vi "Get Angler Position Arrays.vi"(11 "Position Array":T1[](array[typedef])=[{"Angle"=1.0, "Count"=47}, {"Angle"=6.0, "Count"=213}, {"Angle"=5.0, "Count"=383}, {"Angle"=4.0, "Count"=557}, {"Angle"=3.0, "Count"=724}, {"Angle"=2.0, "Count"=898}]) -> (2 "Position Array":i32[](array[numeric]), 3 "Angle Array":dbl[](array[numeric]))   [LabVIEW 2023, in "Angler_ACT.lvlib"]
uses:
  Angler_ACT.lvlib
  Type Defs/Cluster_Angler_Angle to Position.ctl
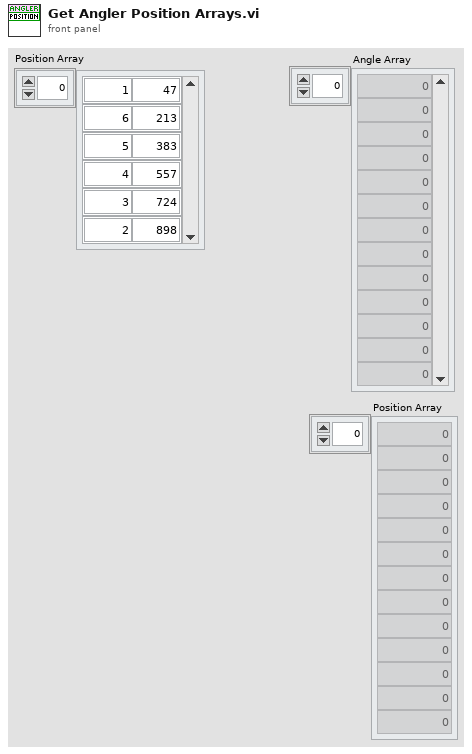
[diagram p1: front panel]
types:
  T1 = typedef "Cluster_Angler_Angle to Position.ctl" = cluster{"Angle":dbl, "Count":i32}
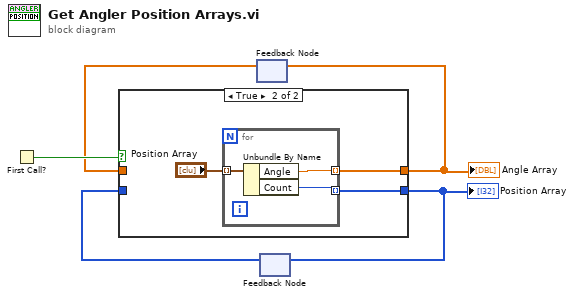
[diagram p0: block diagram]
diagram:
  n1 = First Call?() -> (First Call?: T/F=w5:bool)
  n2 = feedback #1() -> (w2:dbl[])  [unwired: 1 in]
  n3 = feedback #2() -> (w1:i32[])  [unwired: 1 in]
  n4 = case shown="True" w5 {
    tunnel: [w7 w9] -> w4
    tunnel: [w6 w8] -> w3
    tunnel: w2 -> [w7 _]
    tunnel: w1 -> [w6 _]
    frame False {
    }
    frame True {
      n5 = for {
        tunnel: "Position Array" -> [w13] mode=indexing
        tunnel: [w12] -> w9 mode=indexing
        tunnel: [w11] -> w8 mode=indexing
        n6 = Unbundle By Name(w13) -> ("Angle"=w12:dbl, "Count"=w11:i32)
      }
    }
  }
  "Position Array" <- w3
  "Angle Array" <- w4
  n7 = feedback-in #1(w4) -> ()
  n8 = feedback-in #2(w3) -> ()
